vi "Test Move Speed.vi"() -> ()   [LabVIEW 2020]
uses:
  Labview Library/Libraries/HW_PI/E-727/PI E-727 Module/Axis.ctl
  Labview Library/Libraries/HW_PI/E-727/PI E-727 Module/PI E-727 Module.lvlib
panel:
  out "XY Graph":cluster{i32, "Position":dbl}[](graph)=[{0, "Position"=0.009201049805}, {1, "Position"=0.2844314575}, {2, "Position"=2.158081055}, {3, "Position"=3.017997742}, {4, "Position"=54.23788452}, {5, "Position"=12.70572662}, {6, "Position"=130.1732025}, {7, "Position"=145.2370911}, {8, "Position"=122.9711456}, {9, "Position"=104.0599823}, {10, "Position"=72.78260803}, {11, "Position"=88.56982422}, {12, "Position"=72.05151367}, {13, "Position"=128.178894}, {14, "Position"=128.2661591}, {15, "Position"=150.3105469}, {16, "Position"=195.9833984}, {17, "Position"=163.7202454}, {18, "Position"=156.3089142}, {19, "Position"=185.5018616}, {20, "Position"=204.9282532}, {21, "Position"=204.2434082}, {22, "Position"=201.5683899}, {23, "Position"=209.9765472}, {24, "Position"=208.8898621}, {25, "Position"=210.6693726}, {26, "Position"=210.8689117}, {27, "Position"=209.8618622}, {28, "Position"=208.0519104}, {29, "Position"=207.9687195}, {30, "Position"=206.3644257}, {31, "Position"=204.1011658}, {32, "Position"=200.8399506}, {33, "Position"=201.7075195}, {34, "Position"=201.4598389}, {35, "Position"=201.2784729}, {36, "Position"=201.2688599}, {37, "Position"=199.3494415}, {38, "Position"=200.2171783}, {39, "Position"=199.0971375}, {40, "Position"=199.0477753}, {41, "Position"=199.4429626}, {42, "Position"=199.5628815}, {43, "Position"=200.1550293}, {44, "Position"=200.0176544}, {45, "Position"=199.3890076}, {46, "Position"=199.2692413}, {47, "Position"=200.1489563}, {48, "Position"=199.1625977}, {49, "Position"=200.0436096}, {50, "Position"=200.1309814}, {51, "Position"=200.4169464}, {52, "Position"=200.5586548}, {53, "Position"=200.5878906}, {54, "Position"=200.1207275}, {55, "Position"=199.8309021}, {56, "Position"=199.9675903}, {57, "Position"=200.0045929}, {58, "Position"=200.3803711}, {59, "Position"=200.2820129}, {60, "Position"=199.5217743}, {61, "Position"=200.482605}, {62, "Position"=199.705719}, {63, "Position"=200.1302338}, {64, "Position"=200.4356384}, {65, "Position"=199.5124817}, {66, "Position"=200.4127197}, {67, "Position"=200.1460114}, {68, "Position"=199.4688568}, {69, "Position"=200.3482361}, {70, "Position"=199.9266052}, {71, "Position"=199.5210266}, {72, "Position"=200.4057007}, {73, "Position"=200.4292603}, {74, "Position"=200.2229767}, {75, "Position"=200.1182861}, {76, "Position"=200.0879517}, {77, "Position"=200.3269348}, {78, "Position"=200.1242828}, {79, "Position"=200.4677734}, {80, "Position"=200.2889709}, {81, "Position"=200.2192688}, {82, "Position"=199.9496307}, {83, "Position"=199.9141846}, {84, "Position"=199.5904846}, {85, "Position"=199.5916138}, {86, "Position"=200.3955994}, {87, "Position"=199.6832275}, {88, "Position"=200.2133179}, {89, "Position"=199.9865112}, {90, "Position"=199.6660156}, {91, "Position"=200.28683469999999}, {92, "Position"=200.3596649}, {93, "Position"=200.1824341}, {94, "Position"=199.7341461}, {95, "Position"=200.0643616}, {96, "Position"=199.9673462}, {97, "Position"=200.0303345}, {98, "Position"=200.1235962}, {99, "Position"=200.2761841}, {100, "Position"=200.3188629}, {101, "Position"=200.3259888}, {102, "Position"=200.1691895}, {103, "Position"=200.178421}, {104, "Position"=200.0852661}, {105, "Position"=200.2882996}, {106, "Position"=200.3045349}, {107, "Position"=200.2731018}, {108, "Position"=200.0934296}, {109, "Position"=199.8770447}, {110, "Position"=199.8954315}, {111, "Position"=199.7437439}, {112, "Position"=200.2181091}, {113, "Position"=199.759613}, {114, "Position"=199.9078979}, {115, "Position"=199.9414368}, {116, "Position"=200.0389404}]
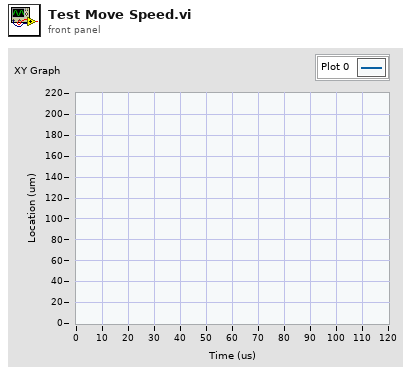
[diagram p1: front panel]
types:
  T1 = typedef "PI E-727 Module.lvlib/Axis.ctl" = enum16{"X", "Y", "Z"}
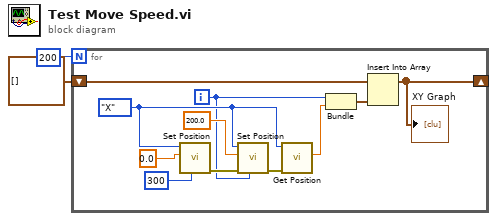
[diagram p0: block diagram]
diagram:
  n1 = for {
    N: 200 -> [_]
    shift-right: [w3] -> _
    shift-left: cluster{i32, "Position":dbl}[] [] -> [w4]
    i -> [w7]
    w12 = Axis."X" ("Axis")
    n2 = call "Set Position.vi"("Idle After Moving (ms)"=300, "Position"=0.0, "Axis"=w12) -> ("error out"=w9:errorcluster)  [unwired: 8 in]
    n3 = call "Set Position.vi"("Idle After Moving (ms)"=w7, "error in"=w9, "Position"=200.0, "Axis"=w12) -> ("error out"=w8:errorcluster)  [unwired: 7 in]
    n4 = call "Get Position.vi"("error in"=w8, "Axis"=w12) -> ("Position"=w6:dbl)  [unwired: 8 in, 1 out]
    n5 = Bundle(w7, "Position"=w6) -> (w5:cluster{i32, "Position":dbl})  [unwired: 1 in]
    n6 = Insert Into Array(array=w4, new element=w5) -> (w3:cluster{i32, "Position":dbl}[])  [unwired: 1 in]
    "XY Graph" <- w3
  }
